vi "Obtain Message Queue.vi"(7 "max queue size (-1, unlimited)":i32=-1 caption="最大队列长度（-1，无限）", 8 "error in (no error)":errorcluster caption="错误输入（无错误）") -> (0 "error out":errorcluster caption="错误输出", 3 "Message Queue":refnum<queue> caption="消息队列")   [LabVIEW 2013, in "Message Queue.lvlib"]
doc: "创建一个队列，数据类型为“消息簇”。"
uses:
  Message Queue.lvlib
  Message Cluster.ctl
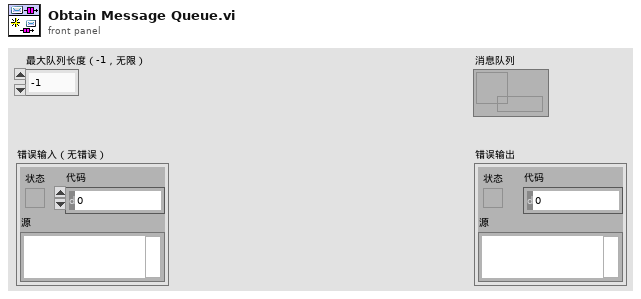
[diagram p1: front panel]
types:
  T1 = typedef "Message Queue.lvlib/Message Cluster.ctl" = cluster{"Message":string, "Message Data":variant}
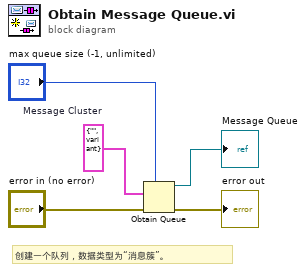
[diagram p0: block diagram]
diagram:
  w5 = T1 {"Message"="", "Message Data"=variant}  # Message Cluster
  # "创建一个队列，数据类型为“消息簇”。"
  n1 = Obtain Queue(max queue size (-1, unlimited)="max queue size (-1, unlimited)", element data type=w5, error in (no error)="error in (no error)") -> (queue out=→"Message Queue":refnum<queue>, error out=→"error out":errorcluster)  [unwired: 2 in, 1 out]
